vi "枚举和下拉列表.vi"() -> ()   [LabVIEW 2018]
panel:
  in  "枚举":enum16{"2000", "1000"}(ring)
  in  "下拉列表":u64(ring) items=["4000"=4000, "3000"=3000, "20M"=2000000, "1000"=1000, ""=4]
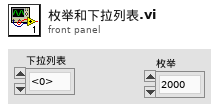
[diagram p1: front panel]
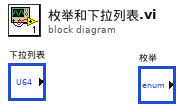
[diagram p0: block diagram]
diagram:
